vi "Read XML_Parse BC Minor Frames.vi"(8 "error in (no error)":errorcluster, 10 "channel in":T1, 11 "busController in":refnum<k24>) -> (0 "error out":errorcluster, 2 "channel out":T1, 3 "busController out":refnum<k24>)   [LabVIEW 2020, in "Ballard 1553 System Explorer.lvlib"]
uses:
  Ballard 1553 System Explorer.lvlib
  Ballard_Channel.ctl
  Ballard_BC.ctl
  Ballard_message.ctl
  Ballard_messageType.ctl
  Ballard_CWD1.ctl
  Ballard_CWD2.ctl
  Ballard_minorFrame.ctl
  Ballard_majorFrame.ctl
  Ballard_acyclicFrame.ctl
  Ballard_RT.ctl
  Ballard_RT subAddress.ctl
  Ballard_RT direction.ctl
  Ballard_RT rtMode.ctl
  Ballard_RT modeCode.ctl
  C:/Users/Administrator/Desktop/GIT/Ballard-MIL-STD-1553-Custom-Device/Source/System Explorer/SubVIs/Parse XML Ballard/1.2/BTIXML_SerDes.dll
  1.2/BTIXML_SerDes.dll
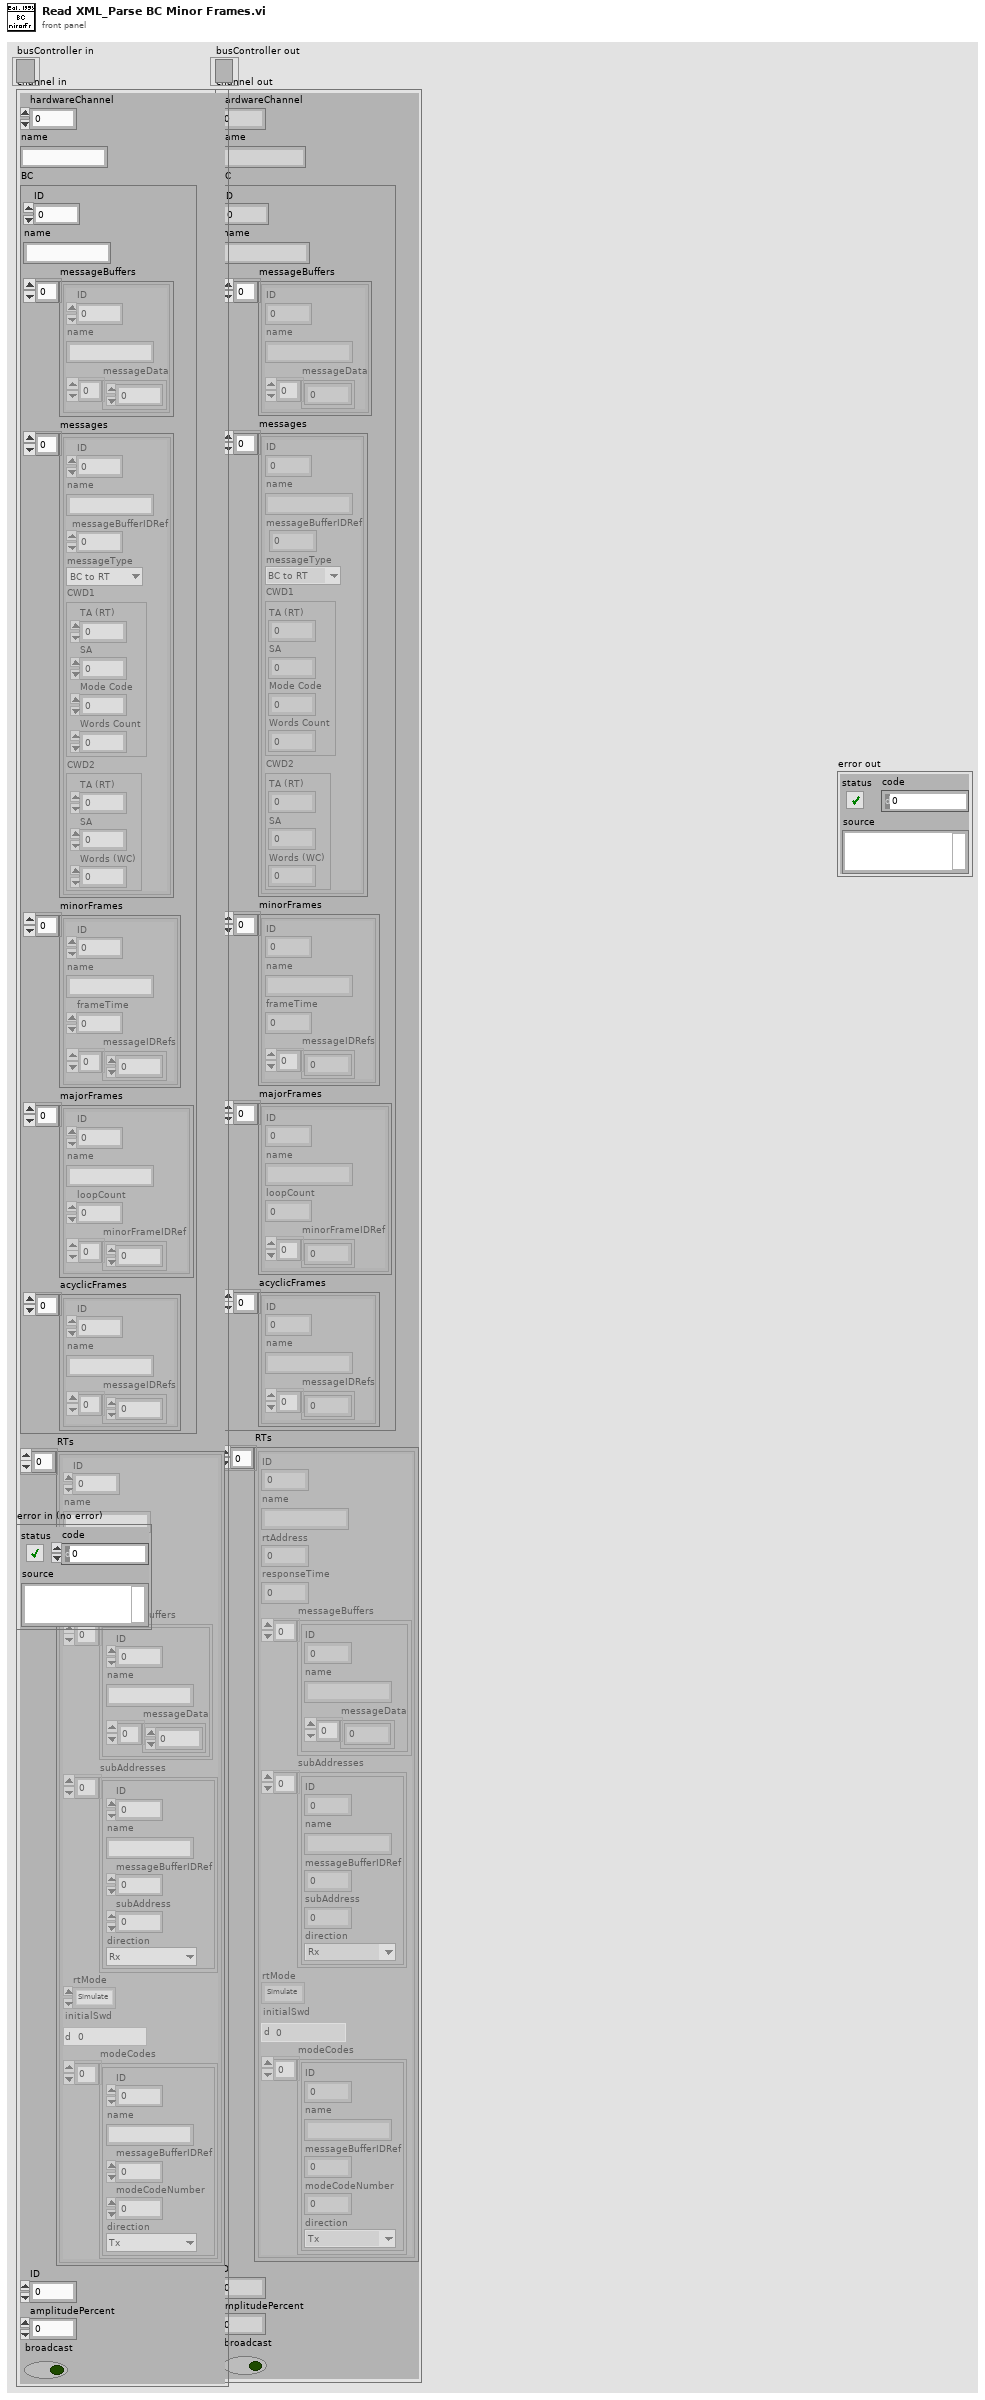
[diagram p1: front panel]
types:
  T1 = typedef "Ballard 1553 System Explorer.lvlib/Ballard_Channel.ctl" = cluster{"hardwareChannel":i32, "name":string, "BC":T2, "RTs":T10[], "ID":i32, "amplitudePercent":dbl, "broadcast":bool}
  T2 = typedef "Ballard 1553 System Explorer.lvlib/Ballard_BC.ctl" = cluster{"ID":i32, "name":string, "messageBuffers":cluster{"ID":i32, "name":string, "messageData":u16[]}[], "messages":T3[], "minorFrames":T7[], "majorFrames":T8[], "acyclicFrames":T9[]}
  T3 = typedef "Ballard 1553 System Explorer.lvlib/Ballard_message.ctl" = cluster{"ID":i32, "name":string, "messageBufferIDRef":i32, "messageType":T4, "CWD1":T5, "CWD2":T6}
  T4 = typedef "Ballard 1553 System Explorer.lvlib/Ballard_messageType.ctl" = enum16{"BC to RT", "RT to BC", "RT to RT", "MC (Rx)", "MC (Tx)"}
  T5 = typedef "Ballard 1553 System Explorer.lvlib/Ballard_CWD1.ctl" = cluster{"TA (RT)":i8, "SA":i8, "Mode Code":i8, "Words Count":i8}
  T6 = typedef "Ballard 1553 System Explorer.lvlib/Ballard_CWD2.ctl" = cluster{"TA (RT)":i8, "SA":i8, "Words (WC)":i8}
  T7 = typedef "Ballard 1553 System Explorer.lvlib/Ballard_minorFrame.ctl" = cluster{"ID":i32, "name":string, "frameTime":i32, "messageIDRefs":i32[]}
  T8 = typedef "Ballard 1553 System Explorer.lvlib/Ballard_majorFrame.ctl" = cluster{"ID":i32, "name":string, "loopCount":i32, "minorFrameIDRef":i32[]}
  T9 = typedef "Ballard 1553 System Explorer.lvlib/Ballard_acyclicFrame.ctl" = cluster{"ID":i32, "name":string, "messageIDRefs":i32[]}
  T10 = typedef "Ballard 1553 System Explorer.lvlib/Ballard_RT.ctl" = cluster{"ID":i32, "name":string, "rtAddress":i8, "responseTime":i32, "messageBuffers":cluster{"ID":i32, "name":string, "messageData":u16[]}[], "subAddresses":T11[], "rtMode":T13, "initialSwd":u16, "modeCodes":T14[]}
  T11 = typedef "Ballard 1553 System Explorer.lvlib/Ballard_RT subAddress.ctl" = cluster{"ID":i32, "name":string, "messageBufferIDRef":i32, "subAddress":i8, "direction":T12}
  T12 = typedef "Ballard 1553 System Explorer.lvlib/Ballard_RT direction.ctl" = enum16{"Tx", "Rx"}
  T13 = typedef "Ballard 1553 System Explorer.lvlib/Ballard_RT rtMode.ctl" = enum16{"Simulate", "Monitor", "Disable"}
  T14 = typedef "Ballard 1553 System Explorer.lvlib/Ballard_RT modeCode.ctl" = cluster{"ID":i32, "name":string, "messageBufferIDRef":i32, "modeCodeNumber":i8, "direction":T12}
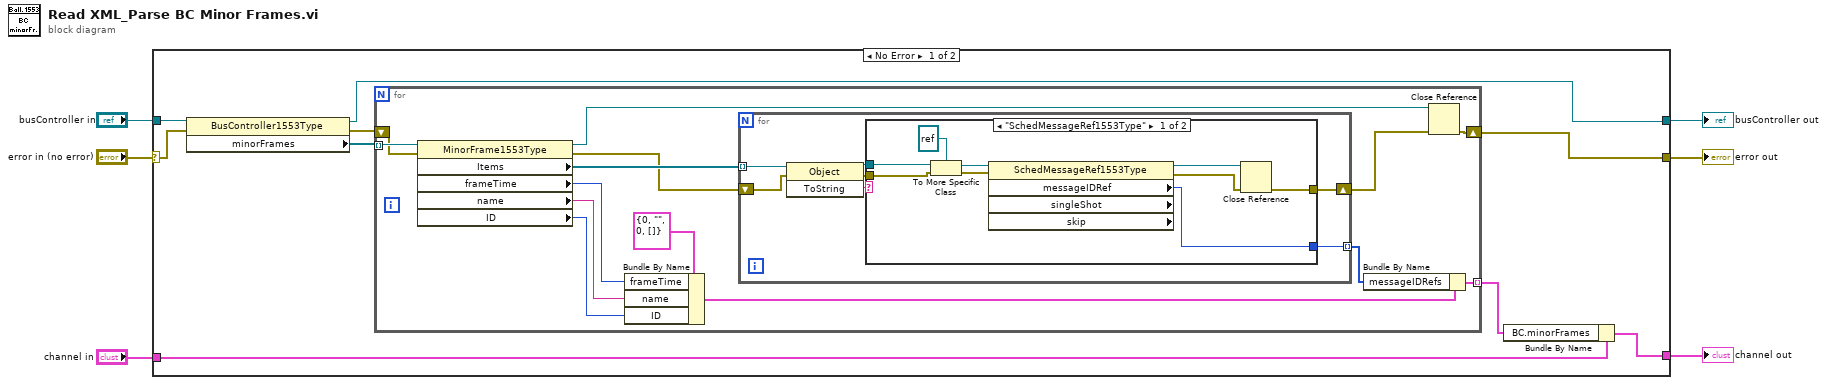
[diagram p0: block diagram]
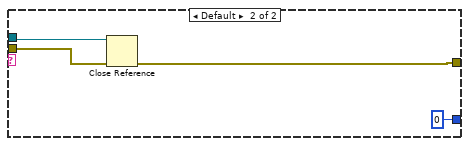
[diagram p2: hidden frame]
diagram:
  n1 = case shown="No Error" "error in (no error)" {
    selector: "error in (no error)" -> [w7 w51]
    tunnel: [w14 w50] -> w6
    tunnel: "channel in" -> [w12 w50]
    tunnel: [w10 w52] -> w4
    tunnel: "busController in" -> [w9 w52]
    tunnel: [w8 w51] -> w2
    frame No Error {
      n2 = property class="BusController1553Type"(reference=w9, error in=w7) -> (reference out=w10:refnum<k24>, error out=w15:errorcluster, "minorFrames"=w11:refnum<k24>[])
      n3 = for {
        tunnel: w11 -> [w29] mode=indexing
        shift-right: [w26] -> w8
        shift-left: w15 -> [w28]
        tunnel: [w16] -> w13 mode=indexing
        n4 = property class="MinorFrame1553Type"(reference=w29, error in=w28) -> (reference out=w27:refnum<k24>, error out=w21:errorcluster, "Items"=w24:refnum<k24>[], "frameTime"=w22:i32, "name"=w23:string, "ID"=w25:i32)
        n5 = Bundle By Name(cluster=T7 {"ID"=0, "name"="", "frameTime"=0, "messageIDRefs"=[]} ("minorFrame"), "frameTime"=w22, "name"=w23, "ID"=w25) -> (w18:T7)
        n6 = for {
          tunnel: w24 -> [w31] mode=indexing
          shift-right: [w32] -> w20
          shift-left: w21 -> [w36]
          tunnel: [w30] -> w17 mode=indexing
          n7 = invoke class="Object" method="ToString"(reference=w31, error in=w36) -> (reference out=w35:refnum<k24>, error out=w34:errorcluster, "ToString"=w33:string)  [unwired: 1 in]
          n8 = case shown="\"SchedMessageRef1553Type\"" w33 {
            tunnel: w35 -> [w45 w49]
            tunnel: w34 -> [w44 w48]
            tunnel: [w39 w47] -> w32
            tunnel: [w38 0 ("messageIDRef")] -> w30
            frame "SchedMessageRef1553Type" {
              n9 = To More Specific Class(target class=refnum<k24> refnum, reference=w45, error in=w44) -> (specific class reference=w42:refnum<k24>, error out=w43:errorcluster)
              n10 = property class="SchedMessageRef1553Type" props=["messageIDRef", "singleShot", "skip"](reference=w42, error in=w43) -> (reference out=w40:refnum<k24>, error out=w41:errorcluster, "messageIDRef"=w38:i32)  [unwired: 2 out]
              n11 = Close Reference(reference=w40, error in (no error)=w41) -> (error out=w39:errorcluster)
            }
            frame Default {
              n12 = Close Reference(reference=w49, error in (no error)=w48) -> (error out=w47:errorcluster)
            }
          }
        }
        n13 = Bundle By Name(cluster=w18, "messageIDRefs"=w17) -> (w16:T7)
        n14 = Close Reference(reference=w27, error in (no error)=w20) -> (error out=w26:errorcluster)
      }
      n15 = Bundle By Name(cluster=w12, "BC.minorFrames"=w13) -> (w14:T1)
    }
    frame Error {
    }
  }
  "channel out" <- w6
  "busController out" <- w4
  "error out" <- w2
